vi "unmap start time tag to channel.vi"(8 "error in (no error)":errorcluster, 11 "References in":T1) -> (0 "error out":errorcluster, 3 "References out":T1)   [LabVIEW 2013, in "Shared Memory editor node.lvclass"]
uses:
  Shared Memory editor node.lvclass
  <vilib>/NI/DCAF/Tag Editor Core/Table API/Table Manager/object ref.ctl
  <vilib>/NI/DCAF/Tag Editor Core/Configuration Editor/Classes/Engine Parent/Engine Parent Editor Node.lvclass
  <vilib>/NI/DCAF/Tag Editor Core/Configuration Editor/Classes/Module editor node/module editor node.lvclass
  <vilib>/NI/Configuration Framework/serializable configuration/NISE_CEF_serializable configuration.lvclass/NISE_CEF_serializable configuration.ctl
  <vilib>/Utility/LVClass/Get LV Class Name.vi
  <vilib>/NI/Configuration Framework/error generator/NISE_error generator.vi
  <vilib>/NI/Configuration Framework/serializable configuration/NISE_CEF_serializable configuration.lvclass
  module/configuration/Shared Memory configuration.lvclass
  <vilib>/NI/Module Execution Interface/Engine Configuration/engine configuration.lvclass
  <vilib>/NI/DCAF/Tag Editor Core/Table API/Table Manager/Table Manager.lvclass
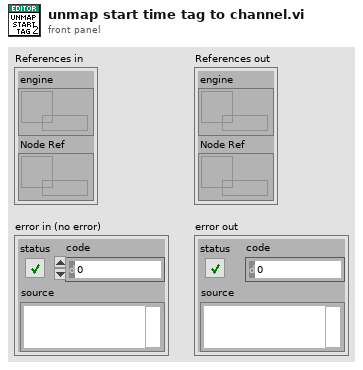
[diagram p1: front panel]
types:
  T1 = typedef "Table Manager.lvlib/Table Manager.lvclass/object ref.ctl" = cluster{"engine":refnum<data-value>, "Node Ref":refnum<data-value>}
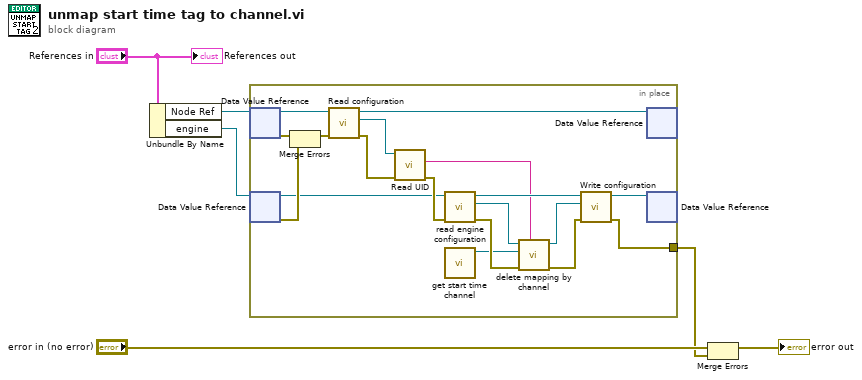
[diagram p0: block diagram]
diagram:
  n1 = Unbundle By Name("References in") -> ("Node Ref"=w3:refnum<data-value>, "engine"=w2:refnum<data-value>)
  n2 = in-place {
    in-place-border: [w13] -> w4
    n3 = in-place-dvr #1(w3) -> (w22:refnum<class "module editor node.lvclass">, w17:errorcluster)
    n4 = in-place-dvr #2(w2) -> (w14:refnum<class "Engine Parent Editor Node.lvclass">, w15:errorcluster)
    n5 = Merge Errors(w17, w15) -> (w16:errorcluster)
    n6 = call-dynamic "Read configuration.vi"("error in"=w16, "NISE_CEF_serializable node in"=w22) -> ("error out"=w21:errorcluster, "configuration"=w19:refnum<class "NISE_CEF_serializable configuration.lvclass">, "NISE_CEF_serializable node out"=w20:refnum<class "module editor node.lvclass">)  [unwired: 7 in]
    n7 = call <vilib>:"Read UID.vi"("error in"=w21, "configuration in"=w19) -> ("error out"=w18:errorcluster, "instance id"=w9:string)  [unwired: 7 in, 1 out]
    n8 = call <vilib>:"read engine configuration.vi"("error in"=w18, "Engine Parent Editor Node in"=w14) -> ("error out"=w8:errorcluster, "engine configuration"=w10:refnum<class "engine configuration.lvclass">, "Engine Parent Editor Node out"=w23:refnum<class "Engine Parent Editor Node.lvclass">)  [unwired: 7 in]
    n9 = call "get start time channel.vi"() -> ("channel"=w7:refnum<class "TBM channel.lvclass">)  [unwired: 11 in]
    n10 = call <vilib>:"delete mapping by channel.vi"("owner ID"=w9, "error in"=w8, "channel"=w7, "engine configuration in"=w10) -> ("error out"=w12:errorcluster, "engine configuration out"=w11:refnum<class "engine configuration.lvclass">)  [unwired: 6 in]
    n11 = call-dynamic "Write configuration.vi"("error in"=w12, "configuration"=w11, "NISE_CEF_serializable node in"=w23) -> ("error out"=w13:errorcluster, "NISE_CEF_serializable node out"=w24:refnum<class "Engine Parent Editor Node.lvclass">)  [unwired: 7 in]
    n12 = in-place-dvr #1(w20) -> ()  [unwired: 2 out]
    n13 = in-place-dvr #2(w24) -> ()  [unwired: 2 out]
  }
  n14 = Merge Errors("error in (no error)", w4) -> (→"error out":errorcluster)
  "References out" <- "References in"
